vi "BRig_dataExp_T_CuePenalty.vi"() -> (2 "output_T_CuePenalty":i32)   [LabVIEW 2014]
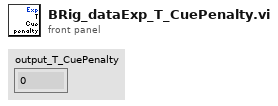
[diagram p1: front panel]
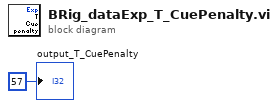
[diagram p0: block diagram]
diagram:
  "output_T_CuePenalty" <- 57 ("output_iBlock")
